vi "parseReportCalibrationDataFrame.vi"(10 "ILCData in":T1 {"Responses"."ReportCalibrationData" items=["OK"=0, "IllegalFunction"=1, "IllegalDataAddress"=2, "IllegalDataValue"=3, "SlaveDeviceFailure"=4, "Acknowledge"=5, "SlaveDeviceBusy"=6, "NegativeAcknowledge"=7, "MemoryParityError"=8, "GatewayPathUnavailable"=9, "GatewayTargetDeviceFailedToRespond"=10, "WaitingForResponse"=254, "CRCError"=255]; "Responses"."ADCOffsetSensitivity" items=["OK"=0, "IllegalFunction"=1, "IllegalDataAddress"=2, "IllegalDataValue"=3, "SlaveDeviceFailure"=4, "Acknowledge"=5, "SlaveDeviceBusy"=6, "NegativeAcknowledge"=7, "MemoryParityError"=8, "GatewayPathUnavailable"=9, "GatewayTargetDeviceFailedToRespond"=10, "WaitingForResponse"=254, "CRCError"=255]; "Responses"."ADCScanRate" items=["OK"=0, "IllegalFunction"=1, "IllegalDataAddress"=2, "IllegalDataValue"=3, "SlaveDeviceFailure"=4, "Acknowledge"=5, "SlaveDeviceBusy"=6, "NegativeAcknowledge"=7, "MemoryParityError"=8, "GatewayPathUnavailable"=9, "GatewayTargetDeviceFailedToRespond"=10, "WaitingForResponse"=254, "CRCError"=255]; "Responses"."Reset" items=["OK"=0, "IllegalFunction"=1, "IllegalDataAddress"=2, "IllegalDataValue"=3, "SlaveDeviceFailure"=4, "Acknowledge"=5, "SlaveDeviceBusy"=6, "NegativeAcknowledge"=7, "MemoryParityError"=8, "GatewayPathUnavailable"=9, "GatewayTargetDeviceFailedToRespond"=10, "WaitingForResponse"=254, "CRCError"=255]; "Responses"."TemporaryAddress" items=["OK"=0, "IllegalFunction"=1, "IllegalDataAddress"=2, "IllegalDataValue"=3, "SlaveDeviceFailure"=4, "Acknowledge"=5, "SlaveDeviceBusy"=6, "NegativeAcknowledge"=7, "MemoryParityError"=8, "GatewayPathUnavailable"=9, "GatewayTargetDeviceFailedToRespond"=10, "WaitingForResponse"=254, "CRCError"=255]; "Responses"."Mode" items=["OK"=0, "IllegalFunction"=1, "IllegalDataAddress"=2, "IllegalDataValue"=3, "SlaveDeviceFailure"=4, "Acknowledge"=5, "SlaveDeviceBusy"=6, "NegativeAcknowledge"=7, "MemoryParityError"=8, "GatewayPathUnavailable"=9, "GatewayTargetDeviceFailedToRespond"=10, "WaitingForResponse"=254, "CRCError"=255]; "Responses"."ReportServerStatus" items=["OK"=0, "IllegalFunction"=1, "IllegalDataAddress"=2, "IllegalDataValue"=3, "SlaveDeviceFailure"=4, "Acknowledge"=5, "SlaveDeviceBusy"=6, "NegativeAcknowledge"=7, "MemoryParityError"=8, "GatewayPathUnavailable"=9, "GatewayTargetDeviceFailedToRespond"=10, "WaitingForResponse"=254, "CRCError"=255]; "Responses"."ReportServerID" items=["OK"=0, "IllegalFunction"=1, "IllegalDataAddress"=2, "IllegalDataValue"=3, "SlaveDeviceFailure"=4, "Acknowledge"=5, "SlaveDeviceBusy"=6, "NegativeAcknowledge"=7, "MemoryParityError"=8, "GatewayPathUnavailable"=9, "GatewayTargetDeviceFailedToRespond"=10, "WaitingForResponse"=254, "CRCError"=255]; "Telemetry"."ADCScanRate" items=["50 Hz"=0, "60 Hz"=1, "100 Hz"=2, "120 Hz"=3, "200 Hz"=4, "240 Hz"=5, "300 Hz"=6, "400 Hz"=7, "480 Hz"=8, "600 Hz"=9, "1200 Hz"=10, "2400 Hz"=11, "4800 Hz"=12, "No Change"=255]; "Command"."ADCScanRate" items=["50 Hz"=0, "60 Hz"=1, "100 Hz"=2, "120 Hz"=3, "200 Hz"=4, "240 Hz"=5, "300 Hz"=6, "400 Hz"=7, "480 Hz"=8, "600 Hz"=9, "1200 Hz"=10, "2400 Hz"=11, "4800 Hz"=12, "No Change"=255]}, 11 "ModbusBuffer in":T10) -> (2 "ILCData out":T1 {"Responses"."ReportCalibrationData" items=["OK"=0, "IllegalFunction"=1, "IllegalDataAddress"=2, "IllegalDataValue"=3, "SlaveDeviceFailure"=4, "Acknowledge"=5, "SlaveDeviceBusy"=6, "NegativeAcknowledge"=7, "MemoryParityError"=8, "GatewayPathUnavailable"=9, "GatewayTargetDeviceFailedToRespond"=10, "WaitingForResponse"=254, "CRCError"=255]; "Responses"."ADCOffsetSensitivity" items=["OK"=0, "IllegalFunction"=1, "IllegalDataAddress"=2, "IllegalDataValue"=3, "SlaveDeviceFailure"=4, "Acknowledge"=5, "SlaveDeviceBusy"=6, "NegativeAcknowledge"=7, "MemoryParityError"=8, "GatewayPathUnavailable"=9, "GatewayTargetDeviceFailedToRespond"=10, "WaitingForResponse"=254, "CRCError"=255]; "Responses"."ADCScanRate" items=["OK"=0, "IllegalFunction"=1, "IllegalDataAddress"=2, "IllegalDataValue"=3, "SlaveDeviceFailure"=4, "Acknowledge"=5, "SlaveDeviceBusy"=6, "NegativeAcknowledge"=7, "MemoryParityError"=8, "GatewayPathUnavailable"=9, "GatewayTargetDeviceFailedToRespond"=10, "WaitingForResponse"=254, "CRCError"=255]; "Responses"."Reset" items=["OK"=0, "IllegalFunction"=1, "IllegalDataAddress"=2, "IllegalDataValue"=3, "SlaveDeviceFailure"=4, "Acknowledge"=5, "SlaveDeviceBusy"=6, "NegativeAcknowledge"=7, "MemoryParityError"=8, "GatewayPathUnavailable"=9, "GatewayTargetDeviceFailedToRespond"=10, "WaitingForResponse"=254, "CRCError"=255]; "Responses"."TemporaryAddress" items=["OK"=0, "IllegalFunction"=1, "IllegalDataAddress"=2, "IllegalDataValue"=3, "SlaveDeviceFailure"=4, "Acknowledge"=5, "SlaveDeviceBusy"=6, "NegativeAcknowledge"=7, "MemoryParityError"=8, "GatewayPathUnavailable"=9, "GatewayTargetDeviceFailedToRespond"=10, "WaitingForResponse"=254, "CRCError"=255]; "Responses"."Mode" items=["OK"=0, "IllegalFunction"=1, "IllegalDataAddress"=2, "IllegalDataValue"=3, "SlaveDeviceFailure"=4, "Acknowledge"=5, "SlaveDeviceBusy"=6, "NegativeAcknowledge"=7, "MemoryParityError"=8, "GatewayPathUnavailable"=9, "GatewayTargetDeviceFailedToRespond"=10, "WaitingForResponse"=254, "CRCError"=255]; "Responses"."ReportServerStatus" items=["OK"=0, "IllegalFunction"=1, "IllegalDataAddress"=2, "IllegalDataValue"=3, "SlaveDeviceFailure"=4, "Acknowledge"=5, "SlaveDeviceBusy"=6, "NegativeAcknowledge"=7, "MemoryParityError"=8, "GatewayPathUnavailable"=9, "GatewayTargetDeviceFailedToRespond"=10, "WaitingForResponse"=254, "CRCError"=255]; "Responses"."ReportServerID" items=["OK"=0, "IllegalFunction"=1, "IllegalDataAddress"=2, "IllegalDataValue"=3, "SlaveDeviceFailure"=4, "Acknowledge"=5, "SlaveDeviceBusy"=6, "NegativeAcknowledge"=7, "MemoryParityError"=8, "GatewayPathUnavailable"=9, "GatewayTargetDeviceFailedToRespond"=10, "WaitingForResponse"=254, "CRCError"=255]; "Telemetry"."ADCScanRate" items=["50 Hz"=0, "60 Hz"=1, "100 Hz"=2, "120 Hz"=3, "200 Hz"=4, "240 Hz"=5, "300 Hz"=6, "400 Hz"=7, "480 Hz"=8, "600 Hz"=9, "1200 Hz"=10, "2400 Hz"=11, "4800 Hz"=12, "No Change"=255]; "Command"."ADCScanRate" items=["50 Hz"=0, "60 Hz"=1, "100 Hz"=2, "120 Hz"=3, "200 Hz"=4, "240 Hz"=5, "300 Hz"=6, "400 Hz"=7, "480 Hz"=8, "600 Hz"=9, "1200 Hz"=10, "2400 Hz"=11, "4800 Hz"=12, "No Change"=255]}, 3 "ModbusBuffer out":T10)   [LabVIEW 2016]
uses:
  Utilities/Modbus/DataTypes/ModbusBuffer.ctl
  DataTypes/ILCData.ctl
  DataTypes/ILCConstants.ctl
  DataTypes/ILCCommand.ctl
  DataTypes/ILCScanRates.ctl
  DataTypes/ILCTelemetry.ctl
  DataTypes/ILCResponses.ctl
  Common_RT_Modbus/DataTypes/ExceptionCodes.ctl
  DataTypes/ILCTimestamps.ctl
  DataTypes/ILCTimings.ctl
  Utilities/Modbus/VIs/ReadU8.vi
  Common_RT_Modbus/RTModbus.lvlib
  Utilities/Modbus/ModbusUtilities.lvlib
  RTILC.lvlib
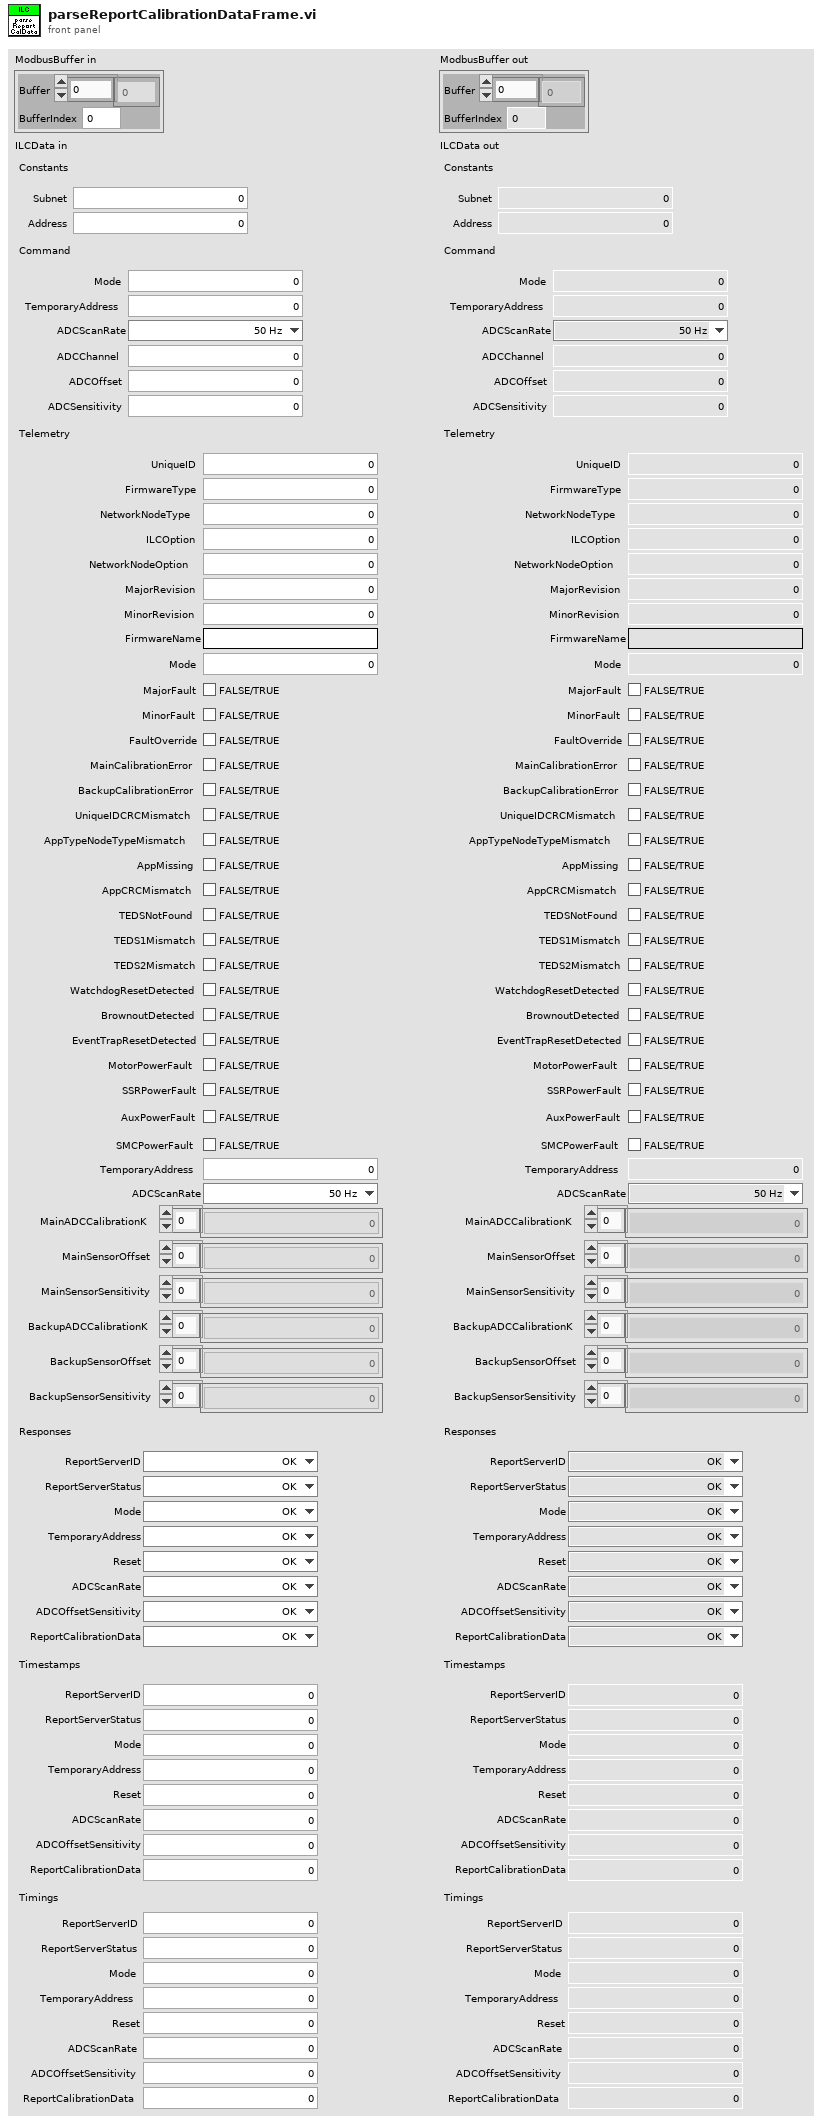
[diagram p1: front panel]
types:
  T1 = typedef "RTILC.lvlib/ILCData.ctl" = cluster{"Constants":T2, "Command":T3, "Telemetry":T5, "Responses":T6, "Timestamps":T8, "Timings":T9}
  T2 = typedef "RTILC.lvlib/ILCConstants.ctl" = cluster{"Subnet":u8, "Address":u8}
  T3 = typedef "RTILC.lvlib/ILCCommand.ctl" = cluster{"Mode":u16, "TemporaryAddress":u8, "ADCScanRate":T4, "ADCChannel":u8, "ADCOffset":sgl, "ADCSensitivity":sgl}
  T4 = typedef "RTILC.lvlib/ILCScanRates.ctl" = u8
  T5 = typedef "RTILC.lvlib/ILCTelemetry.ctl" = cluster{"UniqueID":u64, "FirmwareType":u8, "NetworkNodeType":u8, "ILCOption":u8, "NetworkNodeOption":u8, "MajorRevision":u8, "MinorRevision":u8, "FirmwareName":string, "Mode":u16, "MajorFault":bool, "MinorFault":bool, "FaultOverride":bool, "MainCalibrationError":bool, "BackupCalibrationError":bool, "UniqueIDCRCMismatch":bool, "AppTypeNodeTypeMismatch":bool, "AppMissing":bool, "AppCRCMismatch":bool, "TEDSNotFound":bool, "TEDS1Mismatch":bool, "TEDS2Mismatch":bool, "WatchdogResetDetected":bool, "BrownoutDetected":bool, "EventTrapResetDetected":bool, "MotorPowerFault":bool, "SSRPowerFault":bool, "AuxPowerFault":bool, "SMCPowerFault":bool, "TemporaryAddress":u8, "ADCScanRate":T4, "MainADCCalibrationK":sgl[], "MainSensorOffset":sgl[], "MainSensorSensitivity":sgl[], "BackupADCCalibrationK":sgl[], "BackupSensorOffset":sgl[], "BackupSensorSensitivity":sgl[]}
  T6 = typedef "RTILC.lvlib/ILCResponses.ctl" = cluster{"ReportServerID":T7, "ReportServerStatus":T7, "Mode":T7, "TemporaryAddress":T7, "Reset":T7, "ADCScanRate":T7, "ADCOffsetSensitivity":T7, "ReportCalibrationData":T7}
  T7 = typedef "RTModbus.lvlib/ExceptionCodes.ctl" = u16
  T8 = typedef "RTILC.lvlib/ILCTimestamps.ctl" = cluster{"ReportServerID":dbl, "ReportServerStatus":dbl, "Mode":dbl, "TemporaryAddress":dbl, "Reset":dbl, "ADCScanRate":dbl, "ADCOffsetSensitivity":dbl, "ReportCalibrationData":dbl}
  T9 = typedef "RTILC.lvlib/ILCTimings.ctl" = cluster{"ReportServerID":u32, "ReportServerStatus":u32, "Mode":u32, "TemporaryAddress":u32, "Reset":u32, "ADCScanRate":u32, "ADCOffsetSensitivity":u32, "ReportCalibrationData":u32}
  T10 = typedef "ModbusUtilities.lvlib/ModbusBuffer.ctl" = cluster{"Buffer":u16[], "BufferIndex":i32}
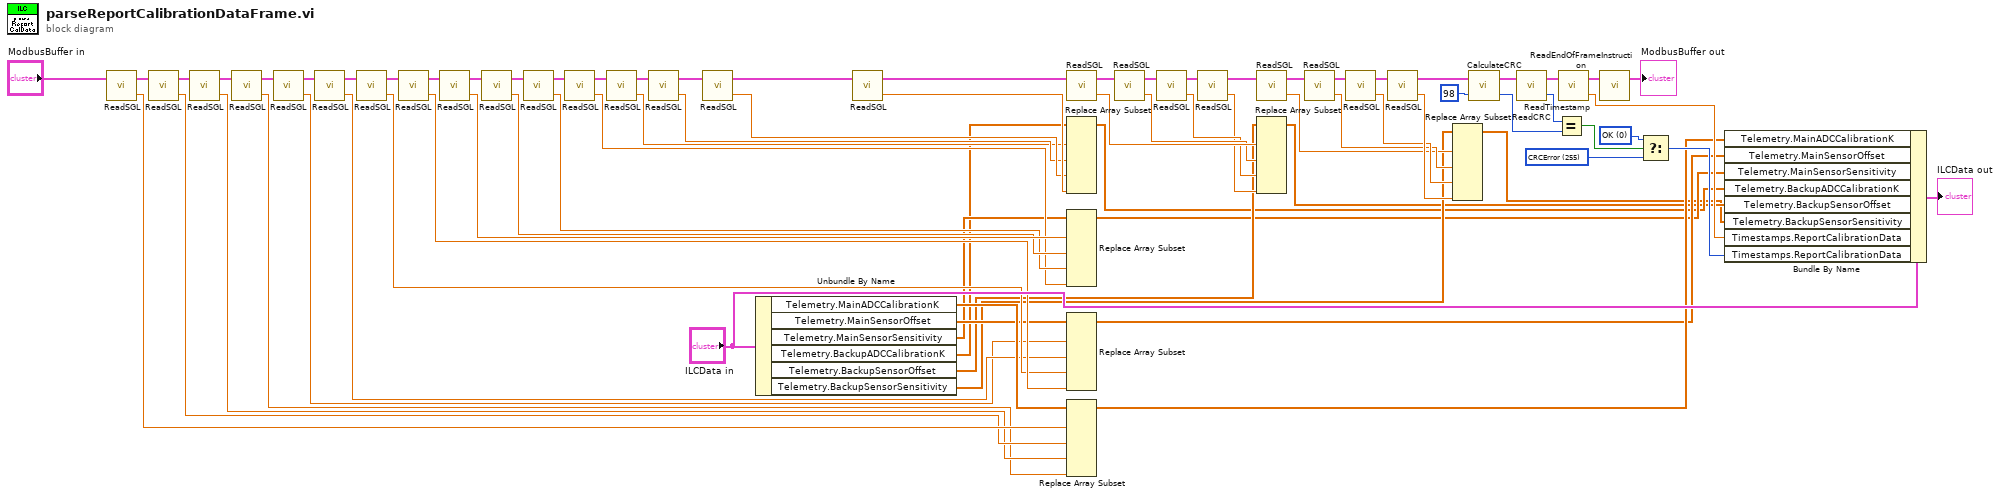
[diagram p0: block diagram]
diagram:
  w65 = T7 255 items=["OK"=0, "IllegalFunction"=1, "IllegalDataAddress"=2, "IllegalDataValue"=3, "SlaveDeviceFailure"=4, "Acknowledge"=5, "SlaveDeviceBusy"=6, "NegativeAcknowledge"=7, "MemoryParityError"=8, "GatewayPathUnavailable"=9, "GatewayTargetDeviceFailedToRespond"=10, "WaitingForResponse"=254, "CRCError"=255] ("f")
  w66 = T7 0 items=["OK"=0, "IllegalFunction"=1, "IllegalDataAddress"=2, "IllegalDataValue"=3, "SlaveDeviceFailure"=4, "Acknowledge"=5, "SlaveDeviceBusy"=6, "NegativeAcknowledge"=7, "MemoryParityError"=8, "GatewayPathUnavailable"=9, "GatewayTargetDeviceFailedToRespond"=10, "WaitingForResponse"=254, "CRCError"=255] ("Responses.ADCOffsetSensitivity")
  n1 = call "ReadSGL.vi"("ModbusBuffer in"="ModbusBuffer in") -> ("Output"=w60:sgl, "ModbusBuffer out"=w55:T10)  [unwired: 1 in]
  n2 = call "ReadSGL.vi"("ModbusBuffer in"=w55) -> ("Output"=w59:sgl, "ModbusBuffer out"=w54:T10)  [unwired: 1 in]
  n3 = call "ReadSGL.vi"("ModbusBuffer in"=w54) -> ("Output"=w58:sgl, "ModbusBuffer out"=w53:T10)  [unwired: 1 in]
  n4 = call "ReadSGL.vi"("ModbusBuffer in"=w53) -> ("Output"=w57:sgl, "ModbusBuffer out"=w17:T10)  [unwired: 1 in]
  n5 = call "ReadSGL.vi"("ModbusBuffer in"=w17) -> ("Output"=w46:sgl, "ModbusBuffer out"=w50:T10)  [unwired: 1 in]
  n6 = call "ReadSGL.vi"("ModbusBuffer in"=w50) -> ("Output"=w47:sgl, "ModbusBuffer out"=w51:T10)  [unwired: 1 in]
  n7 = call "ReadSGL.vi"("ModbusBuffer in"=w51) -> ("Output"=w48:sgl, "ModbusBuffer out"=w52:T10)  [unwired: 1 in]
  n8 = call "ReadSGL.vi"("ModbusBuffer in"=w52) -> ("Output"=w49:sgl, "ModbusBuffer out"=w11:T10)  [unwired: 1 in]
  n9 = call "ReadSGL.vi"("ModbusBuffer in"=w11) -> ("Output"=w45:sgl, "ModbusBuffer out"=w41:T10)  [unwired: 1 in]
  n10 = call "ReadSGL.vi"("ModbusBuffer in"=w41) -> ("Output"=w44:sgl, "ModbusBuffer out"=w40:T10)  [unwired: 1 in]
  n11 = call "ReadSGL.vi"("ModbusBuffer in"=w40) -> ("Output"=w43:sgl, "ModbusBuffer out"=w39:T10)  [unwired: 1 in]
  n12 = call "ReadSGL.vi"("ModbusBuffer in"=w39) -> ("Output"=w42:sgl, "ModbusBuffer out"=w10:T10)  [unwired: 1 in]
  n13 = call "ReadSGL.vi"("ModbusBuffer in"=w10) -> ("Output"=w32:sgl, "ModbusBuffer out"=w36:T10)  [unwired: 1 in]
  n14 = call "ReadSGL.vi"("ModbusBuffer in"=w36) -> ("Output"=w33:sgl, "ModbusBuffer out"=w37:T10)  [unwired: 1 in]
  n15 = call "ReadSGL.vi"("ModbusBuffer in"=w37) -> ("Output"=w34:sgl, "ModbusBuffer out"=w38:T10)  [unwired: 1 in]
  n16 = Unbundle By Name("ILCData in") -> ("Telemetry.MainADCCalibrationK"=w61:sgl[], "Telemetry.MainSensorOffset"=w16:sgl[], "Telemetry.MainSensorSensitivity"=w15:sgl[], "Telemetry.BackupADCCalibrationK"=w14:sgl[], "Telemetry.BackupSensorOffset"=w13:sgl[], "Telemetry.BackupSensorSensitivity"=w12:sgl[])
  n17 = call "ReadSGL.vi"("ModbusBuffer in"=w38) -> ("Output"=w35:sgl, "ModbusBuffer out"=w9:T10)  [unwired: 1 in]
  n18 = call "ReadSGL.vi"("ModbusBuffer in"=w9) -> ("Output"=w31:sgl, "ModbusBuffer out"=w27:T10)  [unwired: 1 in]
  n19 = Replace Array Subset(array=w14, new element #1=w32, new element #2=w33, new element #3=w34, new element #4=w35) -> (w5:sgl[])  [unwired: 4 in]
  n20 = Replace Array Subset(array=w15, new element #1=w45, new element #2=w44, new element #3=w43, new element #4=w42) -> (w6:sgl[])  [unwired: 4 in]
  n21 = Replace Array Subset(array=w16, new element #1=w46, new element #2=w47, new element #3=w48, new element #4=w49) -> (w7:sgl[])  [unwired: 4 in]
  n22 = Replace Array Subset(array=w61, new element #1=w60, new element #2=w59, new element #3=w58, new element #4=w57) -> (w56:sgl[])  [unwired: 4 in]
  n23 = call "ReadSGL.vi"("ModbusBuffer in"=w27) -> ("Output"=w30:sgl, "ModbusBuffer out"=w26:T10)  [unwired: 1 in]
  n24 = call "ReadSGL.vi"("ModbusBuffer in"=w26) -> ("Output"=w29:sgl, "ModbusBuffer out"=w25:T10)  [unwired: 1 in]
  n25 = call "ReadSGL.vi"("ModbusBuffer in"=w25) -> ("Output"=w28:sgl, "ModbusBuffer out"=w8:T10)  [unwired: 1 in]
  n26 = call "ReadSGL.vi"("ModbusBuffer in"=w8) -> ("Output"=w18:sgl, "ModbusBuffer out"=w22:T10)  [unwired: 1 in]
  n27 = Replace Array Subset(array=w13, new element #1=w31, new element #2=w30, new element #3=w29, new element #4=w28) -> (w4:sgl[])  [unwired: 4 in]
  n28 = call "ReadSGL.vi"("ModbusBuffer in"=w22) -> ("Output"=w19:sgl, "ModbusBuffer out"=w23:T10)  [unwired: 1 in]
  n29 = call "ReadSGL.vi"("ModbusBuffer in"=w23) -> ("Output"=w20:sgl, "ModbusBuffer out"=w24:T10)  [unwired: 1 in]
  n30 = call "ReadSGL.vi"("ModbusBuffer in"=w24) -> ("Output"=w21:sgl, "ModbusBuffer out"=w2:T10)  [unwired: 1 in]
  n31 = Replace Array Subset(array=w12, new element #1=w18, new element #2=w19, new element #3=w20, new element #4=w21) -> (w3:sgl[])  [unwired: 4 in]
  n32 = call "CalculateCRC.vi"("Length"=98, "ModbusBuffer in"=w2) -> ("CRC"=w68:u16, "ModbusBuffer out"=w71:T10)
  n33 = call "ReadCRC.vi"("ModbusBuffer in"=w71) -> ("CRC"=w69:u16, "ModbusBuffer out"=w74:T10)  [unwired: 1 in]
  n34 = Equal?(x=w69, y=w68) -> (x = y?=w67:bool)
  n35 = call "ReadTimestamp.vi"("ModbusBuffer in"=w74) -> ("Output"=w63:dbl, "ModbusBuffer out"=w73:T10)  [unwired: 1 in]
  n36 = call "ReadEndOfFrameInstruction.vi"("ModbusBuffer in"=w73) -> ("ModbusBuffer out"=→"ModbusBuffer out":T10)  [unwired: 2 in]
  n37 = Select(t=w66, s=w67, f=w65) -> (s? t:f=w64:T7)
  n38 = Bundle By Name(cluster="ILCData in", "Telemetry.MainADCCalibrationK"=w56, "Telemetry.MainSensorOffset"=w7, "Telemetry.MainSensorSensitivity"=w6, "Telemetry.BackupADCCalibrationK"=w5, "Telemetry.BackupSensorOffset"=w4, "Telemetry.BackupSensorSensitivity"=w3, "Timestamps.ReportCalibrationData"=w63, "Timestamps.ReportCalibrationData"=w64) -> (→"ILCData out":T1)
